vi "Save_Sequence.vi"(0 "Edit_Seq_Array_Input":T3(array[cluster]), 1 "General_Info":T2, 3 "error in (no error)":errorcluster) -> (10 "error out":errorcluster)   [LabVIEW 2023]
doc: "Save Cluster"
panel:
  in  "Sequnce_Info":T1
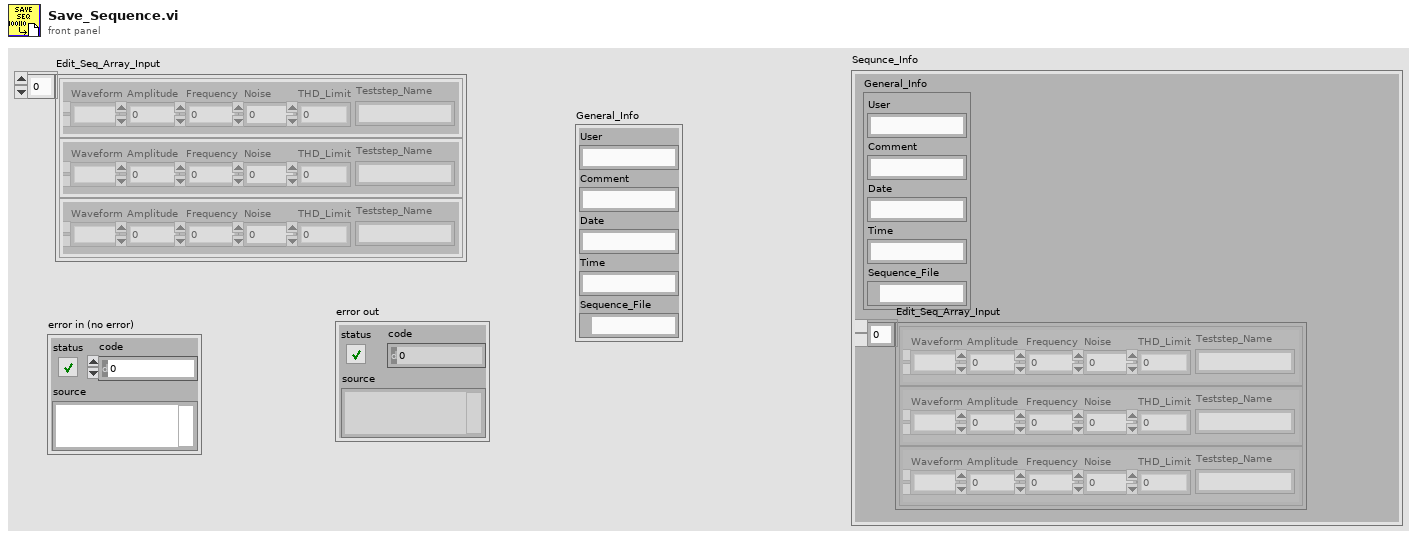
[diagram p1: front panel]
types:
  T1 = cluster{"General_Info":cluster{"User":string, "Comment":string, "Date":string, "Time":string, "Sequence_File":path}, "Edit_Seq_Array_Input":cluster{"Waveform":enum16{"", "Sine Wave", "Triangle Wave", "Square Wave", "Sawtooth Wave"}, "Amplitude":dbl, "Frequency":dbl, "Noise":dbl, "THD_Limit":dbl, "Teststep_Name":string}[]}
  T2 = cluster{"User":string, "Comment":string, "Date":string, "Time":string, "Sequence_File":path}
  T3 = cluster{"Waveform":enum16{"", "Sine Wave", "Triangle Wave", "Square Wave", "Sawtooth Wave"}, "Amplitude":dbl, "Frequency":dbl, "Noise":dbl, "THD_Limit":dbl, "Teststep_Name":string}[]
  T4 = enum16{"open", "replace", "create", "open or create", "replace or create", "replace or create with confirmation"}
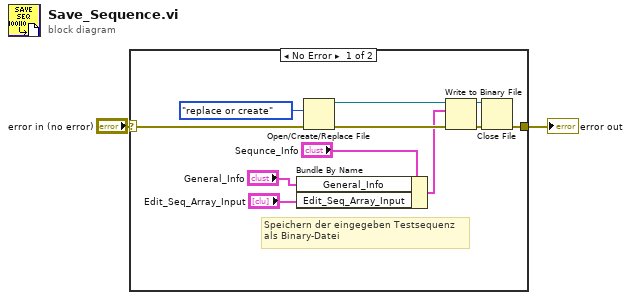
[diagram p0: block diagram]
diagram:
  n1 = case shown="No Error" "error in (no error)" {
    selector: "error in (no error)" -> [w12 w14]
    tunnel: [w11 w14] -> w1
    frame No Error {
      # "Speichern der eingegeben Testsequenz\nals Binary-Datei"
      n2 = Bundle By Name(cluster="Sequnce_Info", "General_Info"="General_Info", "Edit_Seq_Array_Input"="Edit_Seq_Array_Input") -> (w4:T1)
      n3 = Open/Create/Replace File(error in=w12, operation (0:open)=T4."replace or create") -> (refnum out=w8:refnum<file>, error out=w7:errorcluster)  [unwired: 4 in, 1 out]
      n4 = Write to Binary File(file (use dialog)=w8, data=w4, error in=w7) -> (refnum out=w9:refnum<file>, error out=w13:errorcluster)  [unwired: 3 in, 1 out]
      n5 = Close File(refnum=w9, error in=w13) -> (error out=w11:errorcluster)  [unwired: 1 out]
    }
    frame Error {
    }
  }
  "error out" <- w1
